vi "Event Assign Calculator.vi"(6 "Assign Val":string, 8 "Param_Value":dbl[](array[numeric])=[0.35, 180.0, 0.3], 9 "Param_IDs":string[](array[string])=["k1", "k2", "k3", "k4", "C"], 10 "All Variables":string[](array[string]), 11 "transposed array":dbl[][](array[numeric])) -> (2 "y value":dbl format="%.2f")   [LabVIEW 2014]
uses:
  <vilib>/gmath/NI_Gmath.lvlib
panel:
  out "T 2":dbl
  out "T-Sym 2":string="time"
  out "operators (none)":string[](array[string])=["*", "+", "-", "/", "^", "(", ")"]
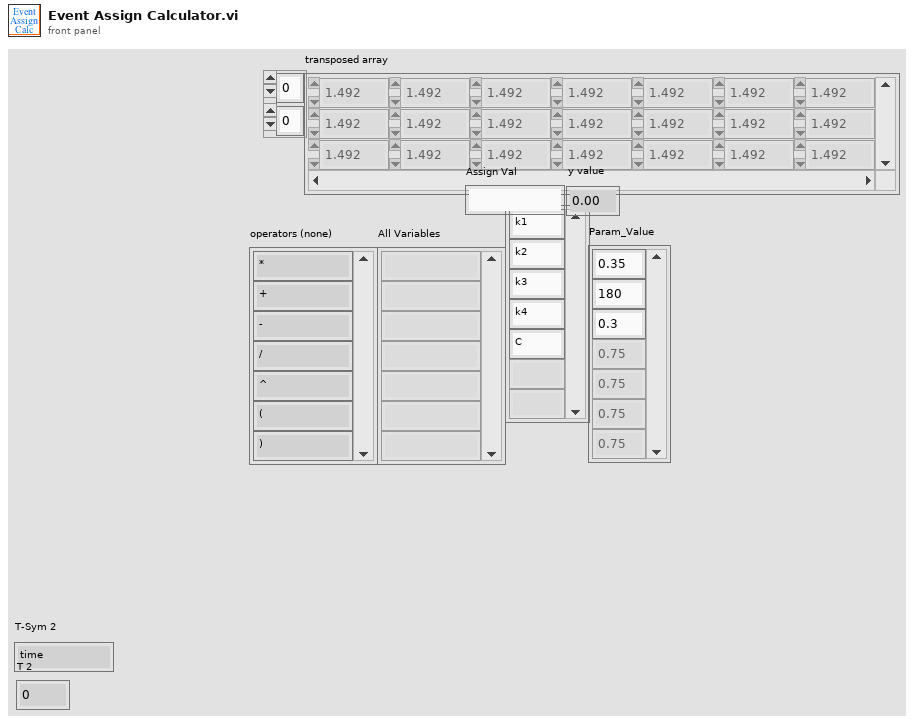
[diagram p1: front panel]
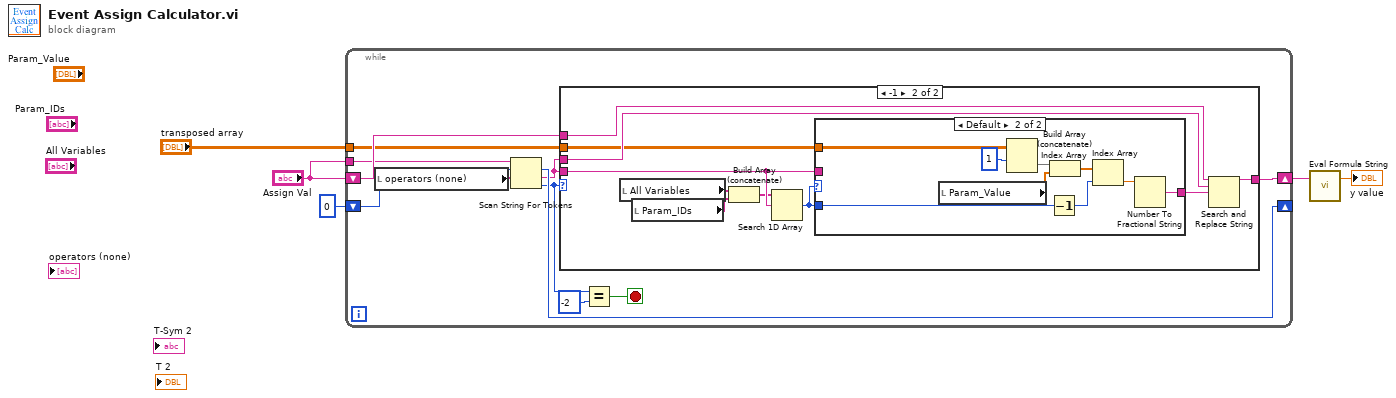
[diagram p0: block diagram]
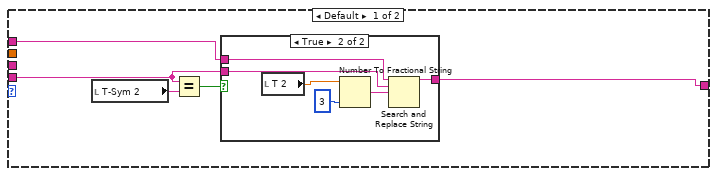
[diagram p2: hidden frame]
diagram:
  n1 = while {
    shift-right: [w13] -> _
    shift-left: 0 ("offset past token") -> [w16]
    shift-right: [w9] -> w2
    shift-left: "Assign Val" -> [w10]
    tunnel: "Assign Val" -> [w7]
    tunnel: "transposed array" -> [w6]
    stop <- w14 stop-if-true
    n2 = local read "operators (none)"() -> (w8:string[])
    n3 = Scan String For Tokens(7:w8, 8:w16, 9:w7) -> (0:w11:i32, 1:w12:string, 2:w13:i32)  [unwired: 3 in, 1 out]
    n4 = case shown="-1" w11 {
      tunnel: w12 -> [w17 w33]
      tunnel: w12 -> [_ w38]
      tunnel: [w20 w36] -> w9
      tunnel: w10 -> [w21 w35]
      tunnel: w6 -> [_ w29]
      frame Default {
        n5 = local read "T-Sym 2"() -> (w19:string)
        n6 = Equal?(x=w17, y=w19) -> (x = y?=w18:bool)
        n7 = case shown="True" w18 {
          tunnel: w21 -> [w22 w28]
          tunnel: [w22 w26] -> w20
          tunnel: w17 -> [_ w24]
          frame False {
          }
          frame True {
            n8 = local read "T 2"() -> (w23:dbl)
            n9 = Number To Fractional String(number=w23, precision (6)=i16 3) -> (F-format string=w27:string)  [unwired: 2 in]
            n10 = Search and Replace String(input string=w28, search string=w24, replace string=w27) -> (result string=w26:string)  [unwired: 5 in, 3 out]
          }
        }
      }
      frame -1 {
        n11 = local read "All Variables"() -> (w31:string[])
        n12 = local read "Param_IDs"() -> (w32:string[])
        n13 = Build Array (concatenate)(w31, w32) -> (w30:string[])
        n14 = Search 1D Array(1D array=w30, element=w33) -> (index of element=w34:i32)  [unwired: 1 in]
        n15 = case shown="Default" w34 {
          tunnel: [w39 w42] -> w37
          tunnel: w34 -> [_ w41]
          tunnel: w33 -> [w39 _]
          tunnel: w29 -> [_ w45]
          frame -1 {
          }
          frame Default {
            n16 = local read "Param_Value"() -> (w46:dbl[])
            n17 = Index Array(array=w45, index (row)=1) -> (element=w47:dbl[])  [unwired: 1 in]
            n18 = Decrement(x=w41) -> (x-1=w40:i32)
            n19 = Build Array (concatenate)(w47, w46) -> (w44:dbl[])
            n20 = Index Array(array=w44, index=w40) -> (element=w43:dbl)
            n21 = Number To Fractional String(number=w43) -> (F-format string=w42:string)  [unwired: 3 in]
          }
        }
        n22 = Search and Replace String(input string=w35, search string=w38, replace string=w37) -> (result string=w36:string)  [unwired: 5 in, 3 out]
      }
    }
    n23 = Equal?(x=w11, y=-2) -> (x = y?=w14:bool)
  }
  n24 = call <vilib>:"Eval Formula String.vi"("formula"=w2) -> ("y value"=→"y value":dbl)  [unwired: 1 in, 1 out]
